vi "zmq atomic counter new.vi"(8 "error in (no error)":errorcluster) -> (0 "error out":errorcluster, 3 "function return":u32)   [LabVIEW 2025, in "LibZMQ.lvlib"]
doc: "ZMQ_EXPORT void *zmq_atomic_counter_new (void);"
uses:
  LibZMQ.lvlib
  LV/LibZMQ/libzmq/lv_x86/bin/Release/libzmq-v143-mt-4_3_6.dll
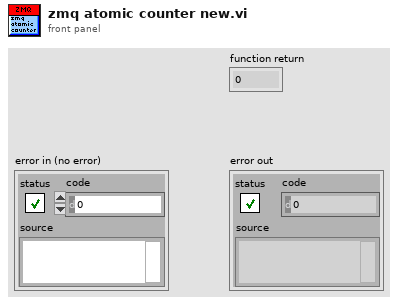
[diagram p1: front panel]
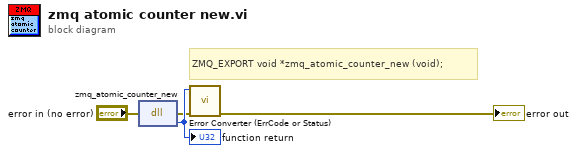
[diagram p0: block diagram]
diagram:
  # "ZMQ_EXPORT void *zmq_atomic_counter_new (void);"
  n1 = dll-call lib="C:/LV/LibZMQ/libzmq/lv_x86/bin/Release/libzmq-v143-mt-4_3_6.*" fn="zmq_atomic_counter_new"(error in="error in (no error)") -> (error out=w2:errorcluster, w4:u32)  [unwired: 2 in, 1 out]
  "function return" <- w4
  n2 = call "Error Converter (ErrCode or Status).vi"("error in (no error)"=w2, "error code"=w4) -> ("error out"=→"error out":errorcluster)  [unwired: 9 in]
